vi "Realtime Clock-DM.vi"(2 "NXT":T3={"Hardware"="NXT", "Flattened String"=""}, 3 "Input Port":T2 items=["Port 1", "Port 2", "Port 3", "Port 4"]) -> (1 "Output of Realtime Clock":T1, 4 "NXT dup":T3={"Hardware"="NXT", "Flattened String"=""} caption="NXT")   [LabVIEW 2010]
uses:
  <vilib>/NXT/Subs/LVHSConnector.ctl
  <vilib>/NXT/Block Support/NXT_InputPort.ctl
  <vilib>/NXT/Block Support/HWPage.SensorType.ctl
  <vilib>/NXT/Block Support/HWPage.SensorMode.ctl
panel:
  # "mindsensors.com\nCopyright (c) 2009 by mindsensors.com\nEmail: info (<at>) mindsensors (<dot>) com\n\nThis program is free software. You can redistribute it and/or modify\nit under the terms of the GNU General Public License as published by\nthe Free Software Foundation; version 3 of the License.\nRead the license at: http://www.gnu.org/licenses/gpl.txt"
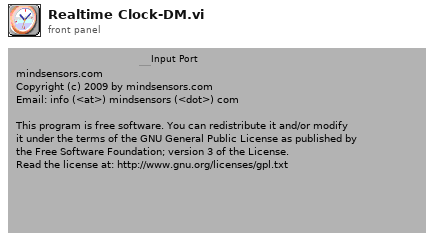
[diagram p1: front panel]
types:
  T1 = cluster{"date string":string, "date":i8, "month":i8, i16, "time string":string, "Hour":i8, "minute":i8, "second":i8}
  T2 = typedef "NXT_InputPort.ctl" = u8
  T3 = typedef "LVHSConnector.ctl" = cluster{"Hardware":string, "Flattened String":string}
  T4 = typedef "HWPage.SensorType.ctl" = u8
  T5 = typedef "HWPage.SensorMode.ctl" = u8
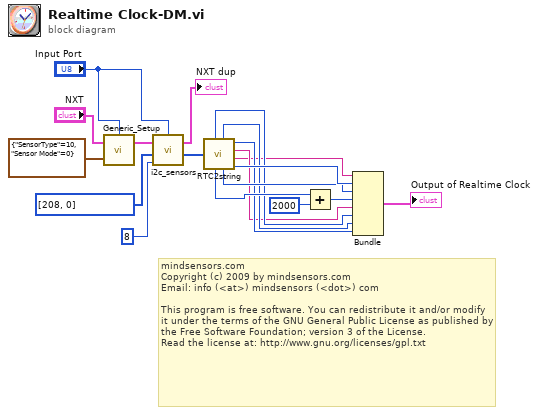
[diagram p0: block diagram]
diagram:
  # "mindsensors.com\nCopyright (c) 2009 by mindsensors.com\nEmail: info (<at>) mindsensors (<dot>) com\n\nThis program is free software. You can redistribute it and/or modify\nit under the terms of the GNU General Public License as published by\nthe Free Software Foundation; version 3 of the License.\nRead the license at: http://www.gnu.org/licenses/gpl.txt"
  n1 = call <vilib>:"Generic_Setup.vi"("Sensor Setup"=cluster{"SensorType":T4, "Sensor Mode":T5} {"SensorType"=10, "Sensor Mode"=0}, "NXT"="NXT", "Port"="Input Port") -> ("NXT"=w16:T3)  [unwired: 1 out]
  n2 = call <vilib>:"i2c_sensors.vi"("Return Length"=8 ("Response Length (0)"), "Bytes to Write"=u8[] [208, 0] ("Buffer"), "NXT"=w16, "Port"="Input Port") -> ("Bytes read"=w14:u8[], "NXT"=→"NXT dup":T3)  [unwired: 1 in, 1 out]
  n3 = call "RTC2string.vi"("array"=w14) -> ("Hour"=w6:i8, "year"=w10:i16, "minute"=w5:i8, "second"=w4:i8, "time string"=w3:string, "month"=w8:i8, "date string"=w2:string, "date"=w9:i8)  [unwired: 1 in, 1 out]
  n4 = Add(x=w10, y=i16 2000) -> (x+y=w7:i16)
  n5 = Bundle("date string"=w2, "date"=w9, "month"=w8, w7, "time string"=w3, "Hour"=w6, "minute"=w5, "second"=w4) -> (→"Output of Realtime Clock":T1)  [unwired: 1 in]
